vi "sourcemeter and signal analyzer.vi"() -> ()   [LabVIEW 2018]
panel:
  in  "Multiplier":dbl=1000000000000.0 format="%#_13e"
  in  "String 3":string="v_dn_21July.lvm"
  out "XY Graph":cluster{"Y":dbl[], "Y":dbl[]}[](graph)
  in  "String 2":string="v_dn_21July.lvm"
  in  "String1":string="N_2205_pressure_"
  in  "File Save Folder":path=path "D:/Soumen/OrbitalShaker/Pressure measurement/2205 particles/Run_21July/heating"
  in  "File save - yes/ no?":bool
  in  "No. of Measurements":i32=1000
  in  "Direction - up (on)/ down(off)":bool=TRUE
  in  "Step":dbl
  in  "End Voltage":dbl
  in  "Start Voltage":dbl
  out "Save File Path":path
  out "Measure loop count":i32
  out "Voltage Loop count":i32
  out "Set Voltage":string
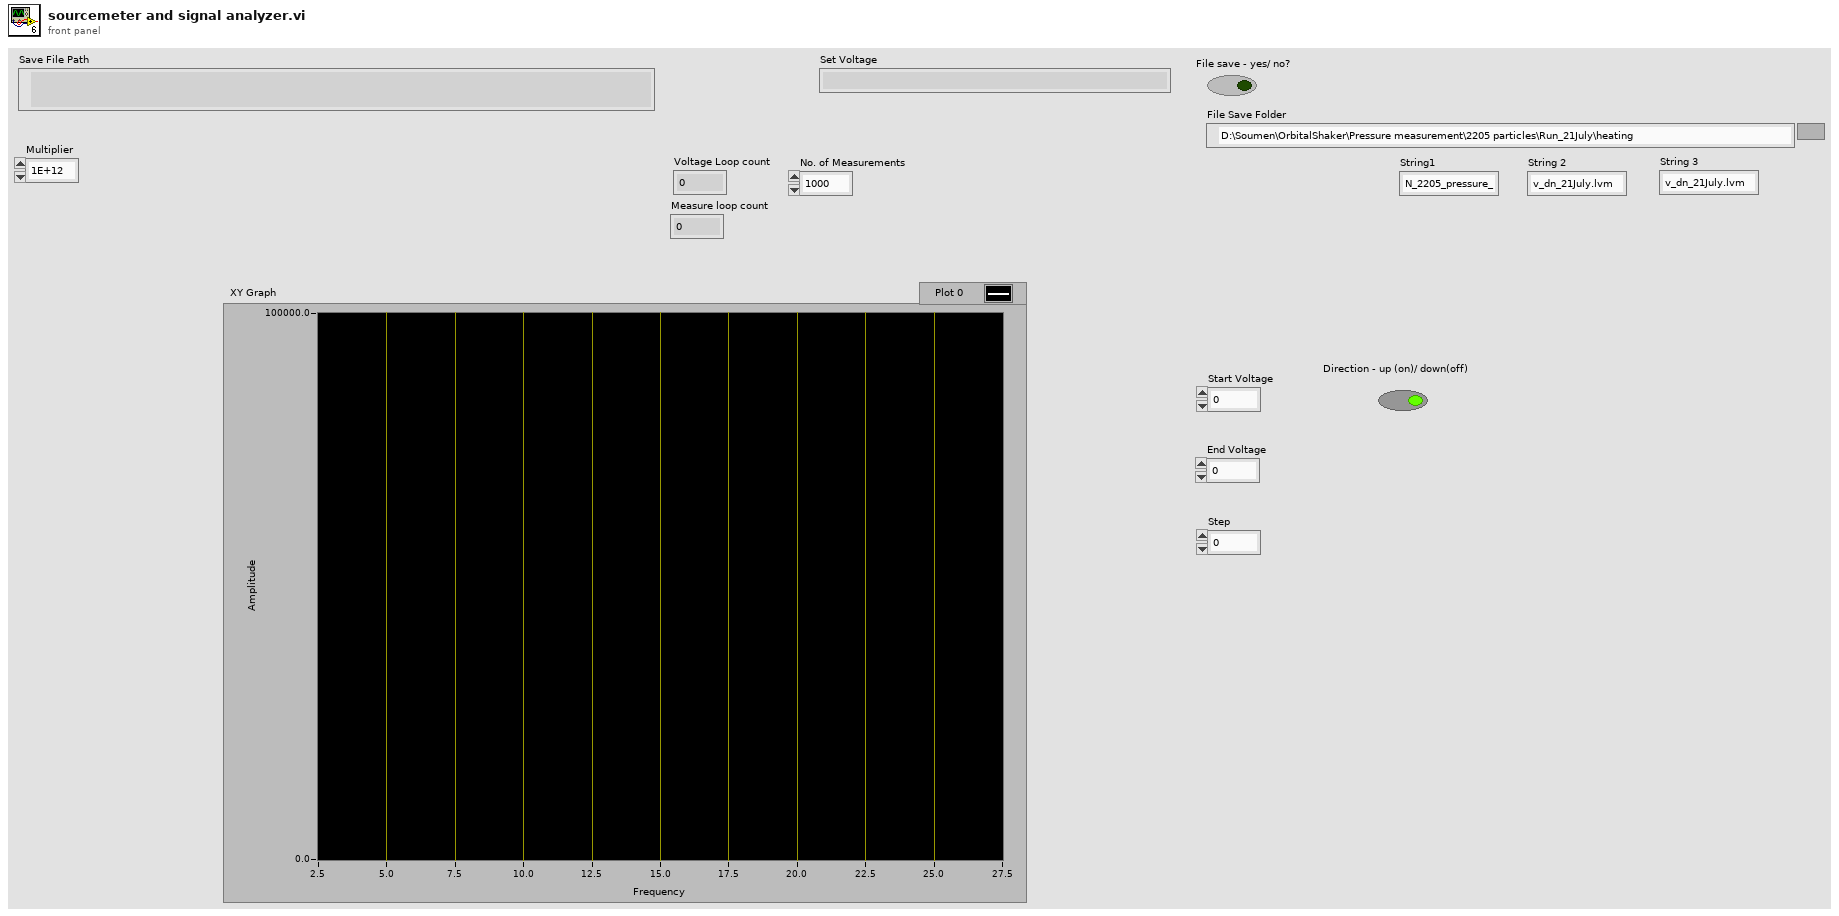
[diagram p1: front panel]
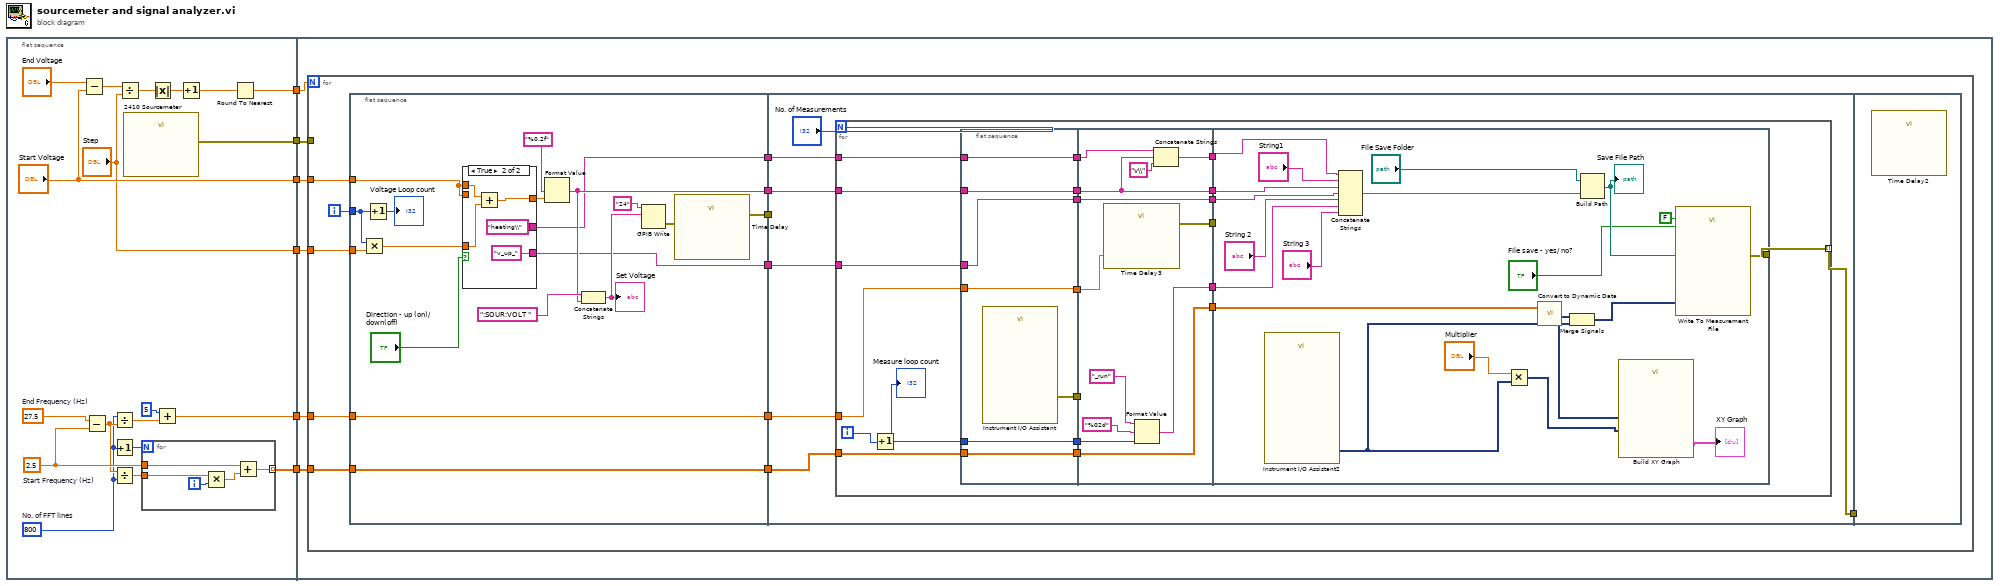
[diagram p0: block diagram]
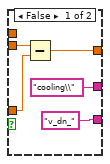
[diagram p2: hidden frame]
diagram:
  n1 = flat-sequence {
    tunnel: [w22] -> w6
    tunnel: ["Start Voltage"] -> w5
    tunnel: ["Step"] -> w4
    tunnel: [w17] -> w3
    tunnel: [w8] -> w2
    tunnel: [w7] -> w1
    tunnel: w6 -> [w36]
    tunnel: w5 -> [w35]
    tunnel: w4 -> [w34]
    tunnel: w3 -> [w33]
    tunnel: w2 -> [w32]
    tunnel: w1 -> [w31]
    frame #0 {
      w16 = 27.5  # End Frequency (Hz)
      w10 = 800  # No. of FFT lines
      w15 = 2.5  # Start Frequency (Hz)
      n2 = Subtract(x="End Voltage", y="Start Voltage") -> (x-y=w24:dbl)
      n3 = Subtract(x=w16, y=w15) -> (x-y=w13:dbl)
      n4 = Divide(x=w10, y=w13) -> (x/y=w12:dbl)
      n5 = Increment(x=w10) -> (x+1=w9:i32)
      n6 = Divide(x=w13, y=w10) -> (x/y=w14:dbl)
      n7 = Divide(x=w24, y="Step") -> (x/y=w19:dbl)
      n8 = call "2410 Sourcemeter"() -> ("error out"=w17:errorcluster)  [unwired: 26 in, 1 out]
      n9 = for {
        N: w9 -> [_]
        tunnel: w15 -> [w30]
        tunnel: w14 -> [w28]
        tunnel: [w26] -> w7 mode=indexing
        i -> [w29]
        n10 = Multiply(x=w28, y=w29) -> (x*y=w27:dbl)
        n11 = Add(x=w30, y=w27) -> (x+y=w26:dbl)
      }
      n12 = Absolute Value(x=w19) -> (abs(x)=w18:dbl)
      n13 = Add(x=5, y=w12) -> (x+y=w8:dbl)
      n14 = Increment(x=w18) -> (x+1=w23:dbl)
      n15 = Round To Nearest(number=w23) -> (nearest integer value=w22:dbl)
    }
    frame #1 {
      n16 = for {
        N: w36 -> [_]
        tunnel: w35 -> [w45]
        tunnel: w34 -> [w44]
        tunnel: w33 -> [_]
        tunnel: w32 -> [w42]
        tunnel: w31 -> [w40]
        i -> [w48]
        n17 = flat-sequence {
          tunnel: w48 -> [w59]
          tunnel: [w61] -> w46
          tunnel: w45 -> [w55]
          tunnel: w44 -> [w60]
          tunnel: [w54] -> w43
          tunnel: w42 -> [w54]
          tunnel: [w53] -> w41
          tunnel: w40 -> [w53]
          tunnel: [w52] -> w39
          tunnel: [w51] -> w38
          tunnel: [w49] -> w37
          tunnel: [w82] -> w47
          tunnel: w46 -> [w81]
          tunnel: w43 -> [w80]
          tunnel: w41 -> [w79]
          tunnel: w39 -> [w78]
          tunnel: w38 -> [w77]
          tunnel: w37 -> [_]
          tunnel: w47 -> [_]
          frame #0 {
            n18 = Multiply(x=w59, y=w60) -> (x*y=w58:dbl)
            n19 = Increment(x=w59) -> (x+1=→"Voltage Loop count":i32)
            n20 = case shown="True" "Direction - up (on)/ down(off)" {
              tunnel: w58 -> [w70 w76]
              tunnel: w55 -> [_ w75]
              tunnel: [w71 w74] -> w56
              tunnel: w55 -> [w69 _]
              tunnel: ["cooling\\" "heating\\"] -> w52
              tunnel: ["v_dn_" "v_up_"] -> w51
              frame False {
                n21 = Subtract(x=w69, y=w70) -> (x-y=w71:dbl)
              }
              frame True {
                n22 = Add(x=w75, y=w76) -> (x+y=w74:dbl)
              }
            }
            n23 = Format Value(format string="%0.2f", value (0)=w56) -> (output string=w61:string)  [unwired: 1 in]
            n24 = Concatenate Strings(":SOUR:VOLT ", w61) -> (w62:string)
            "Set Voltage" <- w62
            n25 = GPIB Write(0:"24" ("address string"), 1:w62) -> (6:w63:errorcluster)  [unwired: 3 in, 1 out]
            n26 = call "Time Delay"("error in (no error)"=w63) -> ("error out"=w49:errorcluster)  [unwired: 10 in]
          }
          frame #1 {
            n27 = for {
              N: "No. of Measurements" -> [_]
              tunnel: [w104] -> w82 mode=indexing
              tunnel: w81 -> [w96]
              tunnel: w80 -> [w102]
              tunnel: w79 -> [w101]
              tunnel: w78 -> [w89]
              tunnel: w77 -> [w87]
              i -> [w95]
              n28 = Increment(x=w95) -> (x+1=w84:i32)
              "Measure loop count" <- w84
              n29 = flat-sequence {
                tunnel: [w111] -> w103
                tunnel: w102 -> [w111]
                tunnel: w101 -> [w110]
                tunnel: [w110] -> w99
                tunnel: [w109] -> w97
                tunnel: w96 -> [w109]
                tunnel: [w108] -> w94
                tunnel: w84 -> [w108]
                tunnel: [w107] -> w91
                tunnel: [w106] -> w90
                tunnel: w89 -> [w106]
                tunnel: [w105] -> w88
                tunnel: w87 -> [w105]
                tunnel: w103 -> [w123]
                tunnel: [w122] -> w100
                tunnel: w99 -> [w122]
                tunnel: [w116] -> w98
                tunnel: w97 -> [w116]
                tunnel: w94 -> [w121]
                tunnel: [w120] -> w93
                tunnel: [w117] -> w92
                tunnel: w91 -> [_]
                tunnel: w90 -> [w114]
                tunnel: w88 -> [w113]
                tunnel: [w113] -> w86
                tunnel: [w112] -> w85
                tunnel: [w143] -> w104
                tunnel: w100 -> [w131]
                tunnel: w98 -> [w124]
                tunnel: w93 -> [w129]
                tunnel: w92 -> [w127]
                tunnel: w86 -> [w125]
                tunnel: w85 -> [_]
                frame #0 {
                  n30 = call "Instrument I/O Assistant"() -> ("error out"=w107:errorcluster)  [unwired: 26 in, 1 out]
                }
                frame #1 {
                  n31 = call "Time Delay3"("Delay Time (s)"=w123) -> ("error out"=w112:errorcluster)  [unwired: 10 in]
                  n32 = Format Value(string ("")="_run" ("format string"), format string="%02d" ("format string 2"), value (0)=w121) -> (output string=w120:string)
                  n33 = Concatenate Strings(w114, w116, "v\\" ("string")) -> (w117:string)
                }
                frame #2 {
                  n34 = call "Instrument I/O Assistant2"() -> ("token"=w134:dynamicdata)  [unwired: 25 in, 2 out]
                  n35 = Concatenate Strings(w127, "String1", w124, w125, "String 2", w129, "String 3") -> (w140:string)
                  n36 = Multiply(x="Multiplier", y=w134) -> (x*y=w132:dynamicdata)
                  n37 = call "Convert to Dynamic Data"("Array"=w131) -> ("Dynamic Data Type"=w128:dynamicdata)  [unwired: 3 in]
                  n38 = Merge Signals(w128, w134) -> (w135:dynamicdata)
                  n39 = Build Path(base path="File Save Folder", name or relative path=w140) -> (appended path=w139:path)
                  "Save File Path" <- w139
                  n40 = call "Build XY Graph"("Y Input"=w132, "X Input"=w128) -> ("XY Graph"=→"XY Graph":cluster{"X":dbl[], "Y":dbl[]}[])  [unwired: 8 in, 1 out]
                  n41 = call "Write To Measurement File"("Signals"=w135, "Reset"=FALSE, "Enable"="File save - yes/ no?", "Filename"=w139) -> ("error out"=w143:errorcluster)  [unwired: 13 in, 2 out]
                }
              }
            }
          }
          frame #2 {
            n42 = call "Time Delay2"() -> ()  [unwired: 11 in, 1 out]
          }
        }
      }
    }
  }
